vi "Callback.vi"(4 "数据":refnum<vi>, 5 "事件数据":cluster{"arg1":refnum<k24>, "arg2":string}, 6 "控件引用":refnum<k24>, 7 "事件通用数据":cluster{"事件源":i32, "事件类型":u32, "时间标识":u32}) -> ()   [LabVIEW 2014]
uses:
  C:/Users/ok/Desktop/LV_HslCommunication/HslCommunication.dll
  HslCommunication.dll
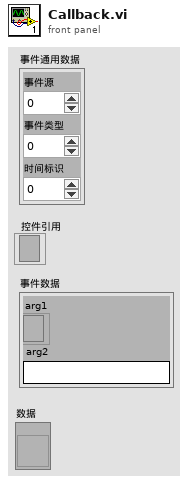
[diagram p1: front panel]
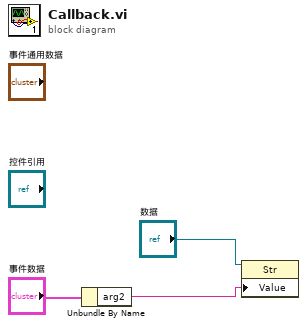
[diagram p0: block diagram]
diagram:
  n1 = Unbundle By Name("事件数据") -> ("arg2"=w1:string)
  n2 = property class="Str"(reference="数据", "Value"=w1) -> ()  [unwired: 1 in, 2 out]
